vi "SEQ Status Json String.vi"() -> ()   [LabVIEW 2017]
uses:
  controls/Seq Status to publish.ctl
  controls/Server CMDs to Publish.ctl
  IPC/MQTT/Controls/MQTT FGV Options.ctl
  support/Message Queue/Auto Message Queue.lvlib
panel:
  out "# elements in queue":i32
  in  "Send":bool
  in  "stop":bool
  out "JSON string":string
  in  "SEQ Status":T1 {"CMD" items=["Display Message", "Step Result", "Aborted", "Log Report", "Traceability", "Vision", "Seq Completed", "Print"]}
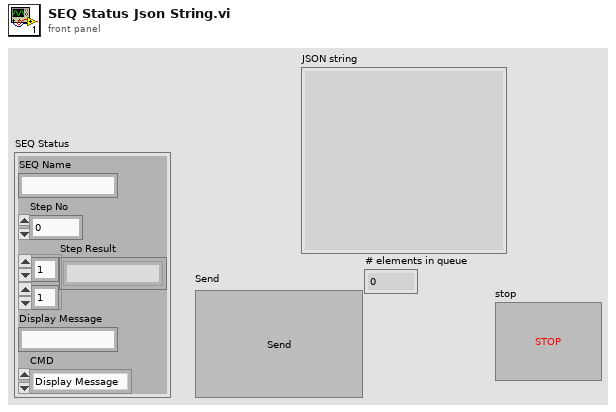
[diagram p1: front panel]
types:
  T1 = typedef "Seq Status to publish.ctl" = cluster{"SEQ Name":string, "Step No":i32, "Step Result":string[][], "Display Message":string, "CMD":T2}
  T2 = typedef "Server CMDs to Publish.ctl" = u16
  T3 = typedef "Auto Message Queue.lvlib/All Message Queues.ctl" = cluster{"UI":refnum<queue>}
  T4 = typedef "MQTT FGV Options.ctl" = enum16{"Read", "Subscribe", "Publish", "Get Status", "Connect", "Disconnect"}
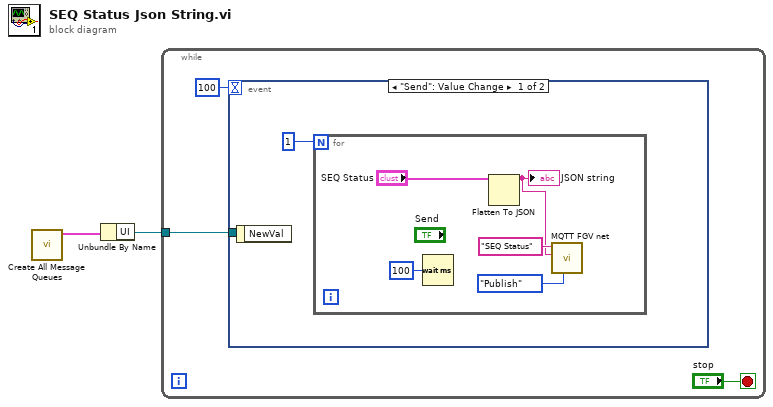
[diagram p0: block diagram]
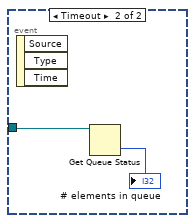
[diagram p2: hidden frame]
diagram:
  n1 = call "Create All Message Queues.vi"() -> ("Message Queues out"=w2:T3)  [unwired: 10 in, 1 out]
  n2 = Unbundle By Name(w2) -> ("UI"=w1:refnum<queue>)
  n3 = while {
    tunnel: w1 -> [w3]
    stop <- "stop" stop-if-true
    n4 = event shown="[0] \"Send\": Value Change" {
      selector: _ -> [_ _]
      dyn-events: _ -> [_ _]
      timeout: 100 -> [_ _]
      tunnel: w3 -> [_ w13]
      event "Send": Value Change {
        n5 = event-data() -> ()  [unwired: 1 in, 1 out]
        n6 = for {
          N: 1 -> [_]
          n7 = Wait (ms)(milliseconds to wait=u32 100) -> ()  [unwired: 1 out]
          n8 = Flatten To JSON(anything="SEQ Status") -> (JSON string=w9:string)  [unwired: 2 in, 1 out]
          "JSON string" <- w9
          n9 = call "MQTT FGV net.vi"("Options"=MQTT_FGV_Options."Publish", "Message"=w9, "Topic"="SEQ Status") -> ()  [unwired: 4 in, 5 out]
        }
      }
      event Timeout {
        n10 = event-data() -> ()  [unwired: 1 in, 3 out]
        n11 = Get Queue Status(queue=w13) -> (# elements in queue=→"# elements in queue":i32)  [unwired: 2 in, 7 out]
      }
    }
  }
